vi "Write Config to File.vi"(8 "error in":errorcluster, 11 "Config":refnum<class "Configuration.lvclass">) -> (0 "error out":errorcluster)   [LabVIEW 2020, in "Configuration.lvclass"]
doc: "Write the configuration to file.\n____\nPeloton Config 2.0.0.9\nCopyright (c) 2024, Peloton"
uses:
  Configuration.lvclass
  C:/Program Files (x86)/National Instruments/LabVIEW 2020/vi.lib/Peloton/Peloton Config/DCFG Framework/Configuration_class/Configuration.lvclass
  <vilib>/Peloton/Peloton Config/DCFG Framework/Configuration_class/Configuration.lvclass/Configuration.ctl
  Configuration.lvclass/Configuration.ctl
  <vilib>/Peloton/Peloton Config/DCFG Framework/Configuration_class/Get File.vi
  Get Configuration.vi
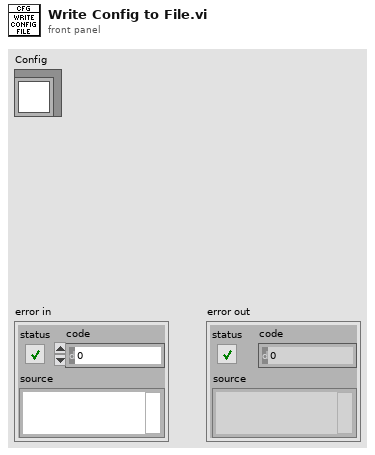
[diagram p1: front panel]
types:
  T1 = typedef "Configuration.lvclass/Configuration--cluster.ctl" = cluster{"a":dbl, "B":dbl}
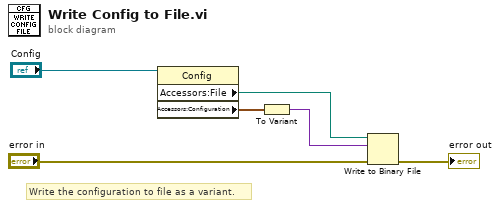
[diagram p0: block diagram]
diagram:
  # "Write the configuration to file as a variant."
  n1 = property class="Config"(reference="Config") -> ("Accessors:File"=w3:path, "Accessors:Configuration"=w2:T1)  [unwired: 1 in, 2 out]
  n2 = To Variant(anything=w2) -> (Variant=w1:variant)
  n3 = Write to Binary File(file (use dialog)=w3, data=w1, error in="error in") -> (error out=→"error out":errorcluster)  [unwired: 3 in, 2 out]
